vi "168xBSetVoltage.vi"() -> ()   [LabVIEW 2017]
uses:
  <vilib>/Instr/_visa.llb/VISA Configure Serial Port (Instr).vi
panel:
  in  "Voltage":sgl min=0 max=30 step=0.1
  out "read buffer 3":string
  out "read buffer 2":string
  out "read buffer":string
  out "error out":errorcluster
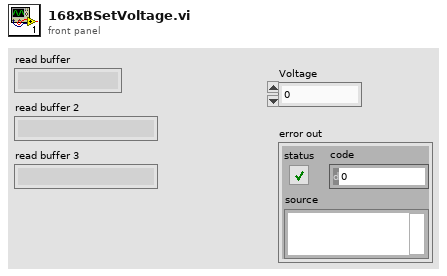
[diagram p1: front panel]
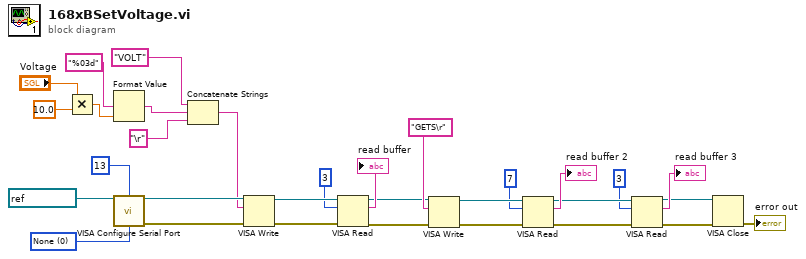
[diagram p0: block diagram]
diagram:
  w29 = u16 0 items=["None", "XON/XOFF", "RTS/CTS", "XON/XOFF & RTS/CTS", "DTR/DSR", "XON/XOFF & DTR/DSR"] ("flow control (0:none)")
  n1 = Multiply(x="Voltage", y=sgl 10.0) -> (x*y=w3:sgl)
  n2 = Format Value(format string="%03d", value (0)=w3) -> (output string=w2:string)  [unwired: 1 in]
  n3 = call-poly "VISA Configure Serial Port"("VISA resource name"=refnum<visa-resource-name> "COM15", "termination char\n(0xA = '\\n' = LF)"=u8 13 ("termination char\n(0xA = '\\n' = LF)"), "flow control (0:none)"=w29) -> ("VISA resource name out"=w16:refnum<visa-resource-name>, "error out"=w15:errorcluster)  [unwired: 11 in]
  n4 = Concatenate Strings("VOLT" ("write buffer"), w2, "\r" ("string")) -> (w6:string)
  n5 = VISA Write(VISA resource name=w16, write buffer=w6, error in (no error)=w15) -> (VISA resource name out=w27:refnum<visa-resource-name>, error out=w28:errorcluster)  [unwired: 1 out]
  n6 = VISA Read(VISA resource name=w27, byte count=u32 3, error in (no error)=w28) -> (VISA resource name out=w19:refnum<visa-resource-name>, read buffer=→"read buffer":string, error out=w18:errorcluster)  [unwired: 1 out]
  n7 = VISA Write(VISA resource name=w19, write buffer="GETS\r", error in (no error)=w18) -> (VISA resource name out=w22:refnum<visa-resource-name>, error out=w23:errorcluster)  [unwired: 1 out]
  n8 = VISA Read(VISA resource name=w22, byte count=u32 7, error in (no error)=w23) -> (VISA resource name out=w10:refnum<visa-resource-name>, read buffer=→"read buffer 2":string, error out=w11:errorcluster)  [unwired: 1 out]
  n9 = VISA Read(VISA resource name=w10, byte count=u32 3, error in (no error)=w11) -> (VISA resource name out=w13:refnum<visa-resource-name>, read buffer=→"read buffer 3":string, error out=w12:errorcluster)  [unwired: 1 out]
  n10 = VISA Close(VISA resource name=w13, error in (no error)=w12) -> (error out=→"error out":errorcluster)
